vi "读取生产统计数据.vi"(8 "线号显示":i32=1, 9 "产品码":string) -> (3 "线号":i32)   [LabVIEW 2014]
uses:
  Controls/MsgAction.ctl
  Global.vi
  <vilib>/Utility/config.llb/Read Key (String).vi
  <vilib>/Utility/config.llb/NI_LVConfig.lvlib
panel:
  out "File out":path
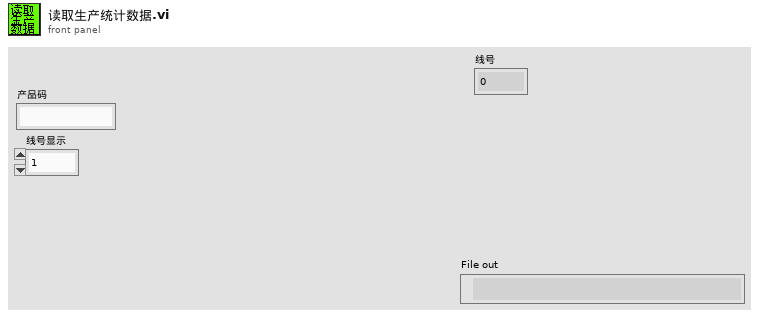
[diagram p1: front panel]
types:
  T1 = typedef "MsgAction.ctl" = enum16{"初始化", "添加消息", "区分结果添加消息", "清空消息", "获取消息"}
  T2 = typedef "NI_LVConfig.lvlib/Config Data RefNum.ctl" = refnum<k1>
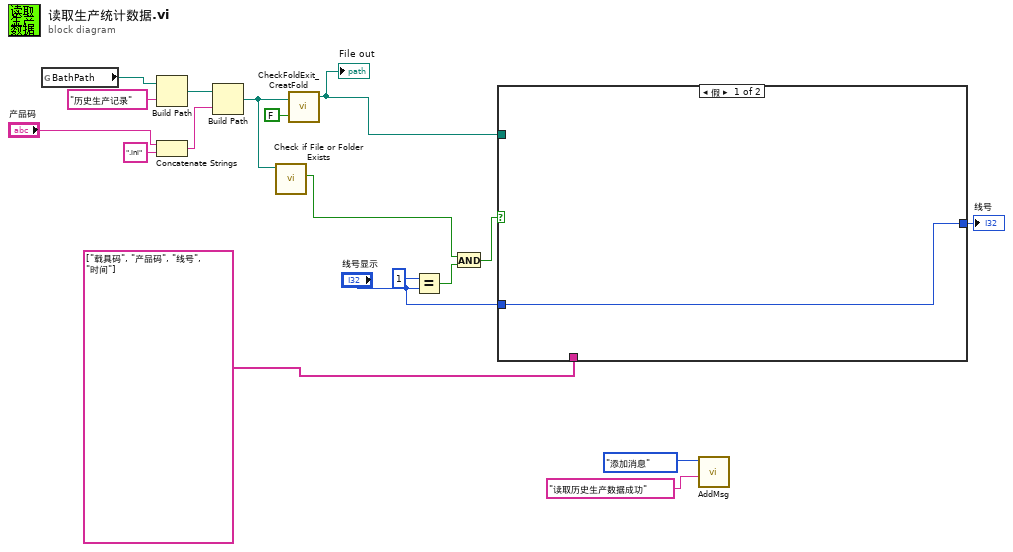
[diagram p0: block diagram]
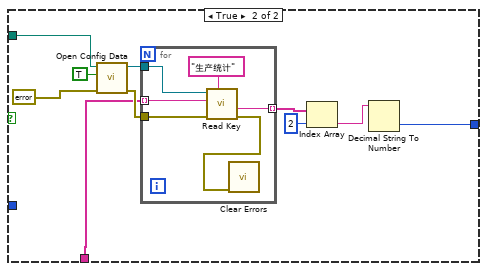
[diagram p2: hidden frame]
diagram:
  n1 = global read "Global.vi" "BathPath"() -> (w12:path)
  n2 = Build Path(base path=w12, name or relative path="历史生产记录" ("名称或相对路径")) -> (appended path=w13:path)
  n3 = Concatenate Strings("产品码", ".ini" ("字符串")) -> (w9:string)
  n4 = Build Path(base path=w13, name or relative path=w9) -> (appended path=w6:path)
  n5 = call <vilib>:"Check if File or Folder Exists.vi"("path"=w6) -> ("file or folder exists?"=w5:bool)  [unwired: 1 in, 9 out]
  n6 = call "CheckFoldExit_CreatFold.vi"("path in"=w6, "FoldOrFile¡H"=FALSE) -> ("File out"=w17:path)  [unwired: 2 out]
  "File out" <- w17
  n7 = Equal?(x=1, y="线号显示") -> (x = y?=w4:bool)
  n8 = And(x=w5, y=w4) -> (x .and. y?=w3:bool)
  n9 = case shown="假" w3 {
    tunnel: w17 -> [_ w28]
    tunnel: [w19 w20] -> w8
    tunnel: string[] ["载具码", "产品码", "线号", "时间"] -> [_ w21]
    tunnel: "线号显示" -> [w19 _]
    frame False {
    }
    frame True {
      n10 = call <vilib>:"Open Config Data.vi"("error in (no error)"=errorcluster {"status"=FALSE, "code"=0, "source"=""} ("error out"), "create file if necessary (T)"=TRUE, "configuration file path"=w28) -> ("error out"=w24:errorcluster, "refnum"=w27:T2)  [unwired: 6 in, 1 out]
      n11 = for {
        tunnel: w27 -> [w35]
        tunnel: w21 -> [w33] mode=indexing
        tunnel: [w32] -> w25 mode=indexing
        tunnel: w24 -> [w31]
        n12 = call-poly <vilib>:"Read Key.vi"("section"="生产统计", "error in (no error)"=w31, "key"=w33, "refnum"=w35) -> ("error out"=w30:errorcluster, "value"=w32:string)  [unwired: 4 in, 2 out]
        n13 = call <vilib>:"Clear Errors.vi"("error in (no error)"=w30) -> ()  [unwired: 5 in, 2 out]
      }
      n14 = Index Array(array=w25, index=2 ("索引")) -> (element=w22:string)
      n15 = Decimal String To Number(string=w22) -> (number=w20:i32)  [unwired: 2 in, 1 out]
    }
  }
  "线号" <- w8
  n16 = call "AddMsg.vi"("添加消息"="读取历史生产数据成功" ("消息显示"), "消息Action"=MsgAction."添加消息") -> ()  [unwired: 2 in, 1 out]
